vi "App_ShowAppInfo_SplashScreen.vi"() -> ()   [LabVIEW 2014]
panel:
  out "FileDescription":string
  out "LegalCopyright":string
  out "CompanyName":string
  out "InternalName":string
  out "ProductName":string
  out "FileVersion":string
  in  "Close":bool
  # "Application Info"
  # "Version:"
  # "Productname:"
  # "Copyright:"
  # "Company:"
  # "Internal Info:"
  # "FileVersion:"
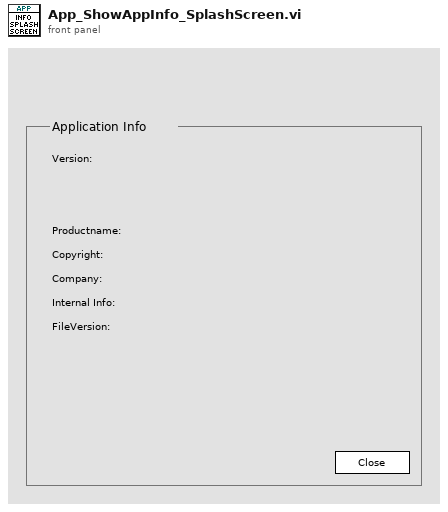
[diagram p1: front panel]
types:
  T1 = enum32{"invalid app kind", "Development System", "Run Time System", "Student Edition", "Embedded LabVIEW", "Evaluation", "Custom"}
  T2 = enum32{"Invalid", "Standard", "Closed", "Hidden", "Minimized", "Maximized"}
  T3 = cluster{"Core":cluster{"Current VI Reference":refnum<vi>, "Close Panel on Exit?":bool}, "Your Boolean data":bool, "Your string data":string}
  T4 = cluster{"Current VI Reference":refnum<vi>, "Close Panel on Exit?":bool}
  T5 = typedef "FileVersionInformation.ctl" = cluster{"FileVersion":string, "ProductName":string, "InternalName":string, "CompanyName":string, "LegalCopyright":string, "FileDescription":string}
  T6 = typedef "SVN_Info_Cluster.ctl" = cluster{"entry.path":string, "entry.revision (HEAD)":i32, "entry.kind":string, "SVN_Log_Cluster":T7}
  T7 = typedef "SVN_LogEntry_Cluster.ctl" = cluster{"revision":i32, "Author":string, "Datetime":timestamp, "Message":string}
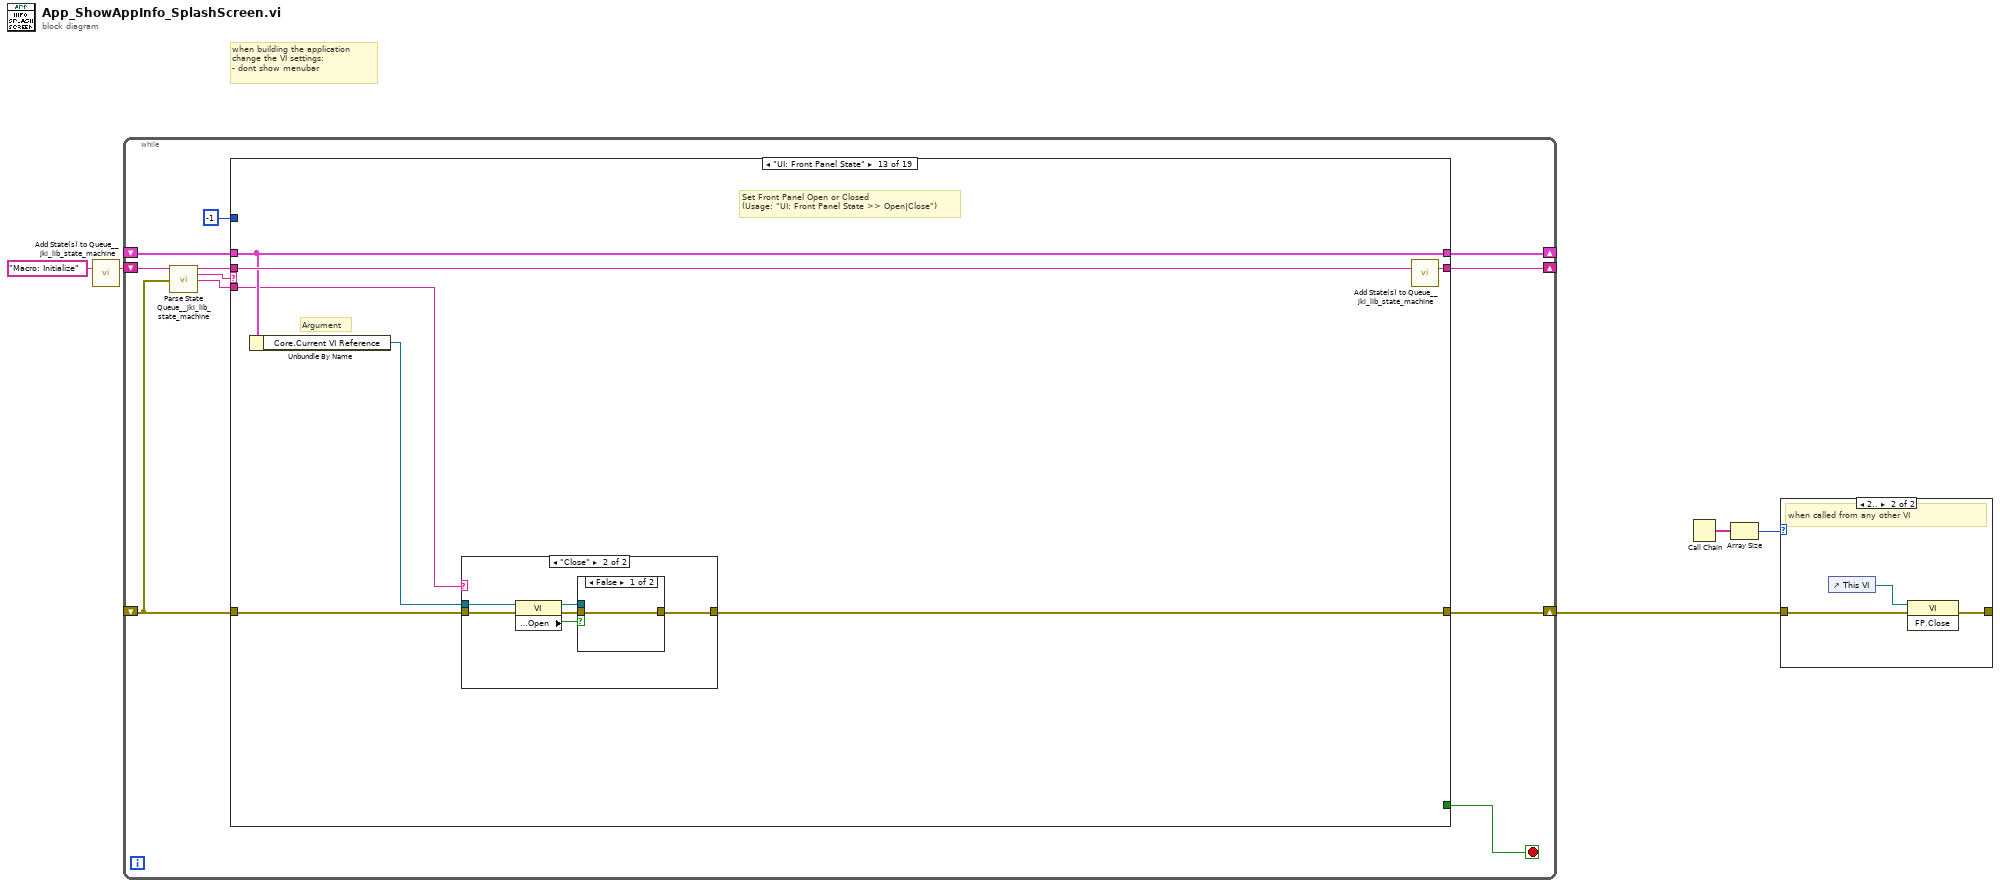
[diagram p0: block diagram]
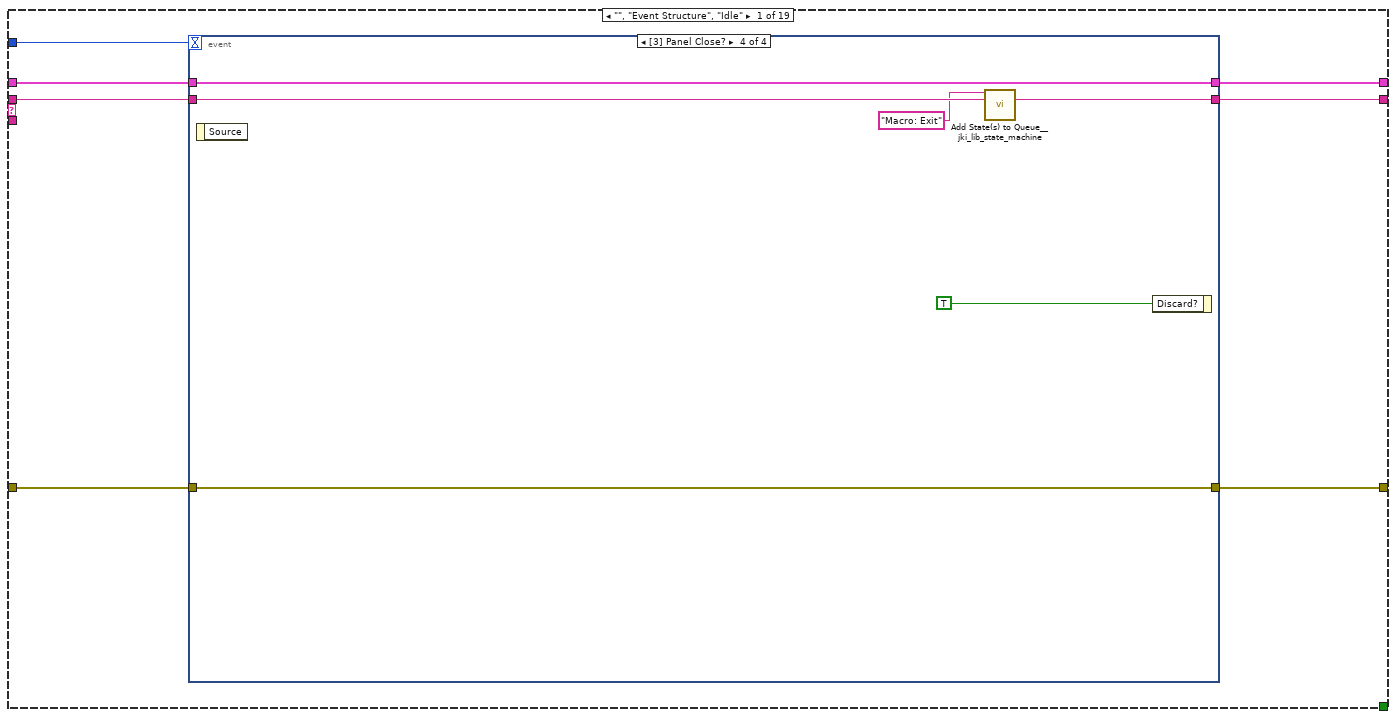
[diagram p3: hidden frame]
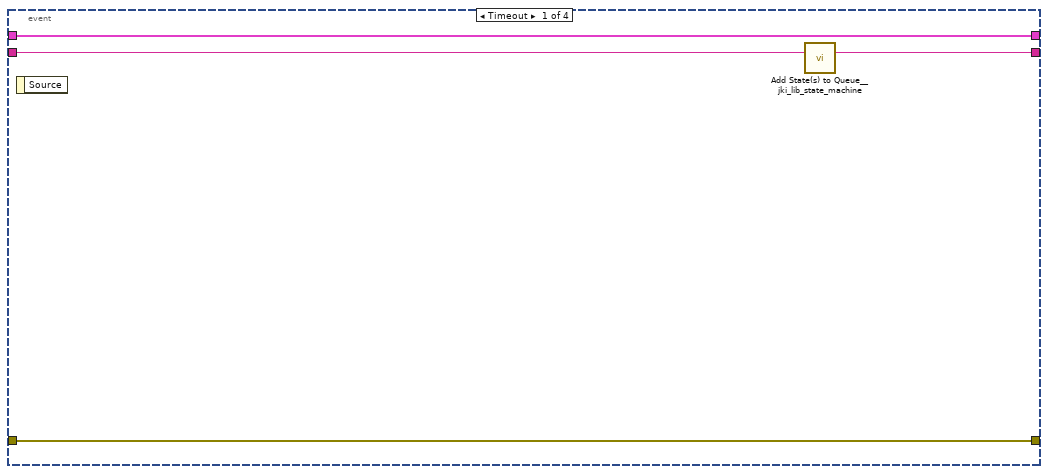
[diagram p4: hidden frame]
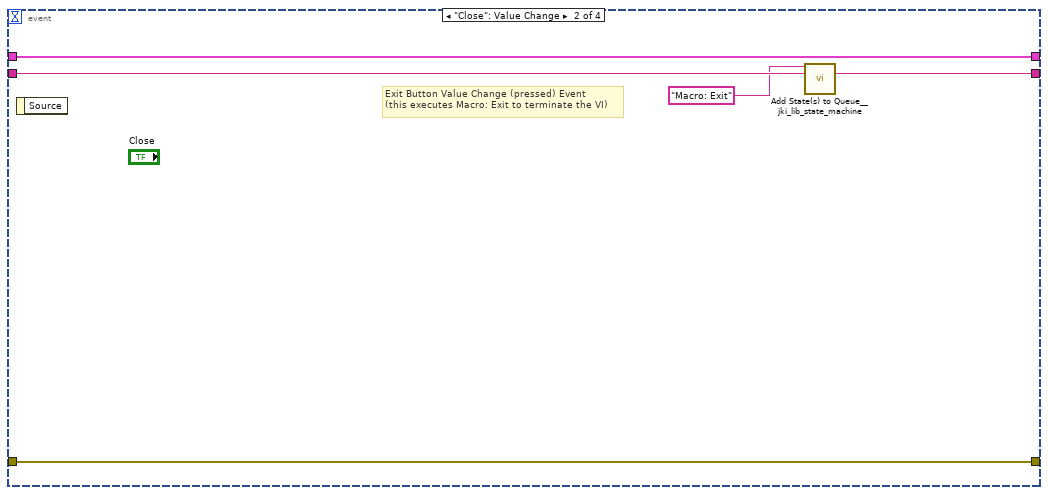
[diagram p5: hidden frame]
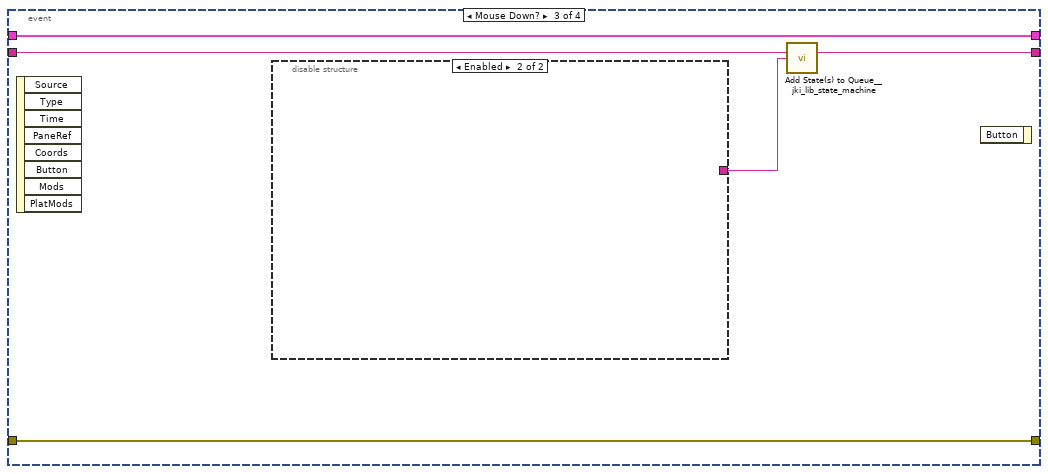
[diagram p6: hidden frame]
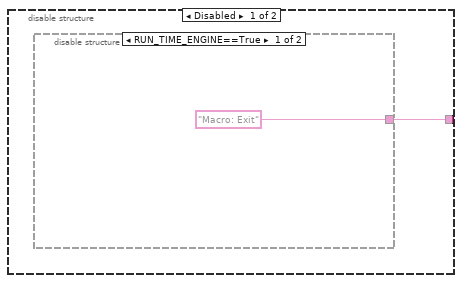
[diagram p7: hidden frame]
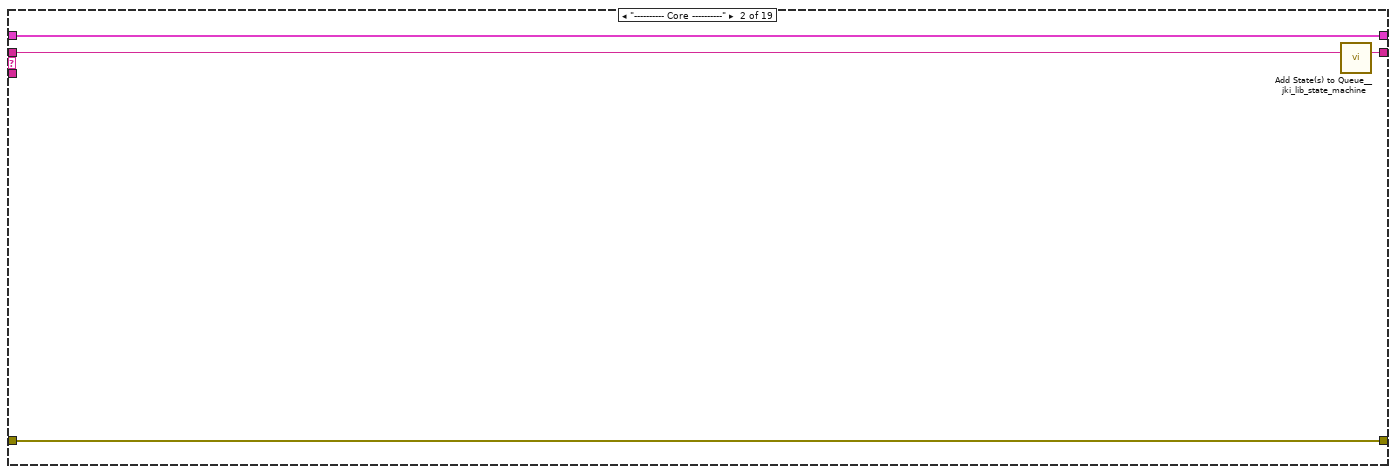
[diagram p9: hidden frame]
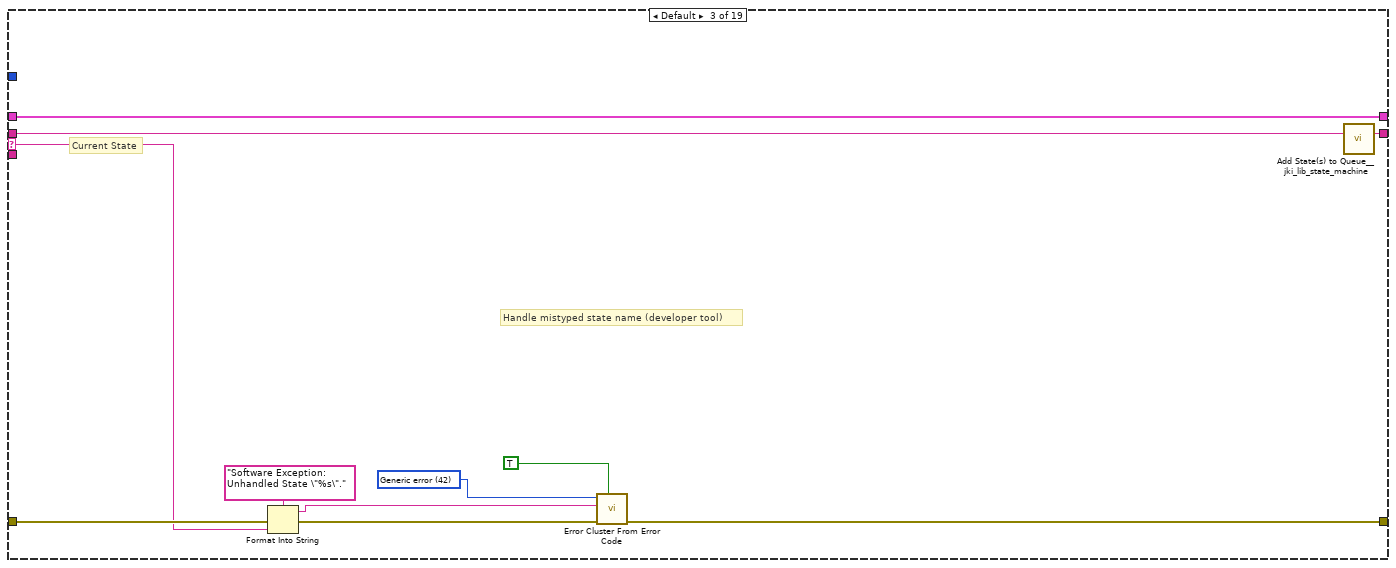
[diagram p10: hidden frame]
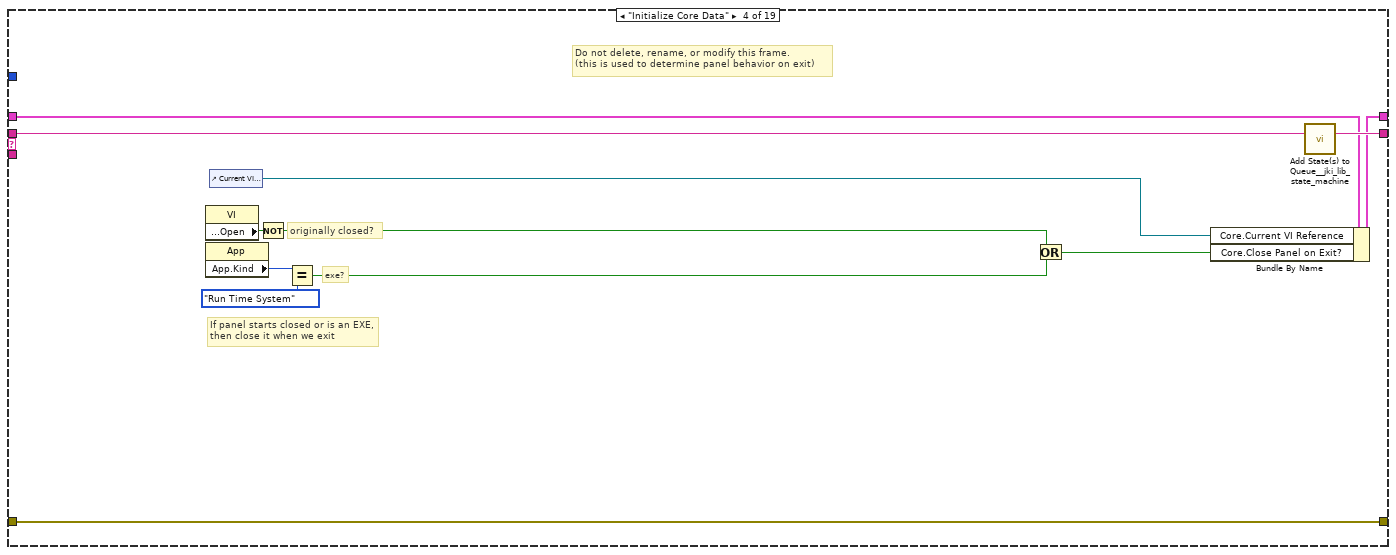
[diagram p11: hidden frame]
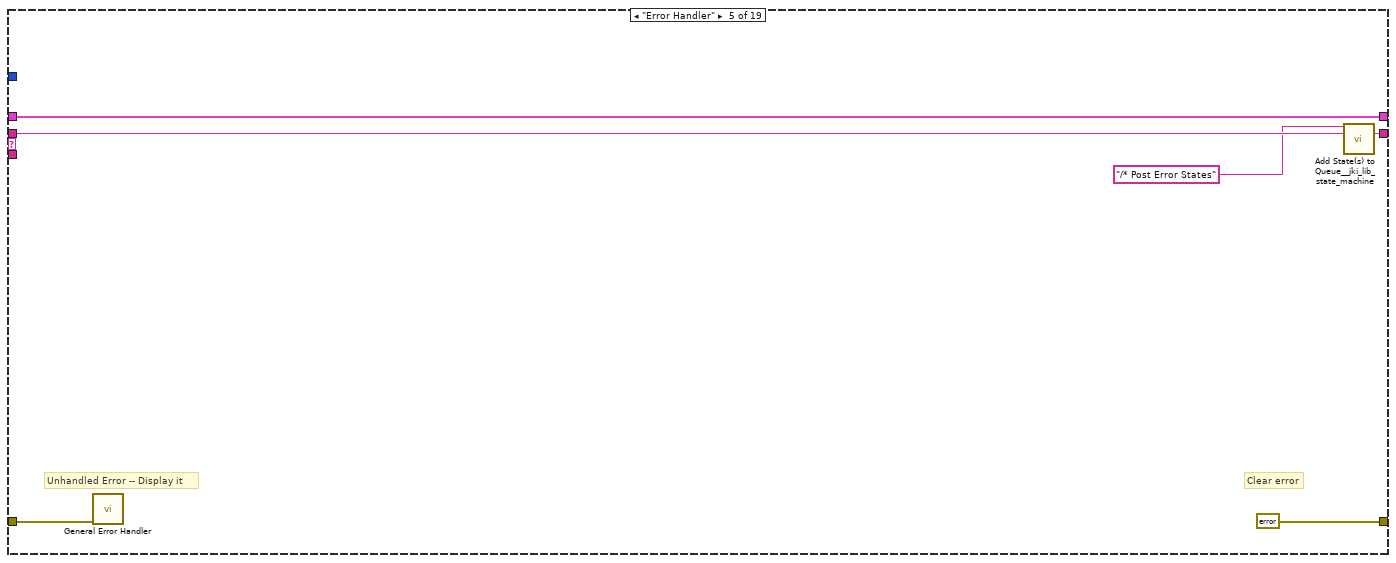
[diagram p12: hidden frame]
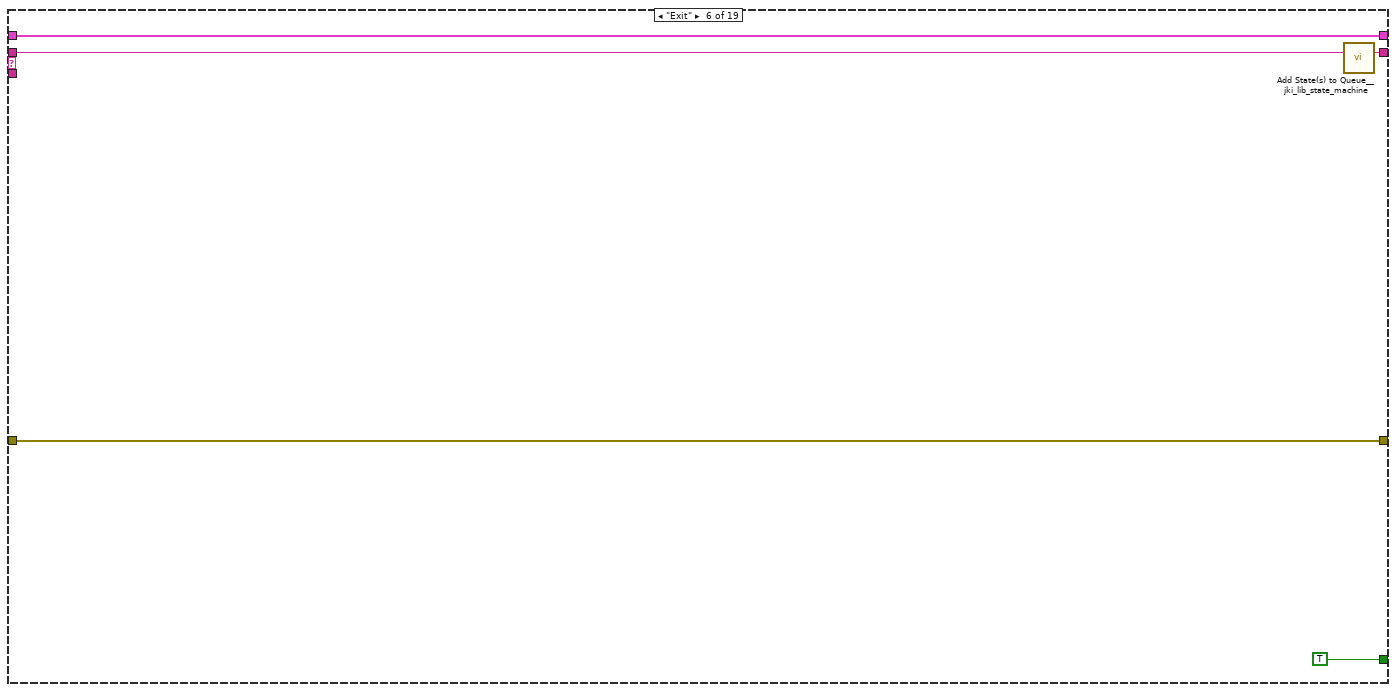
[diagram p13: hidden frame]
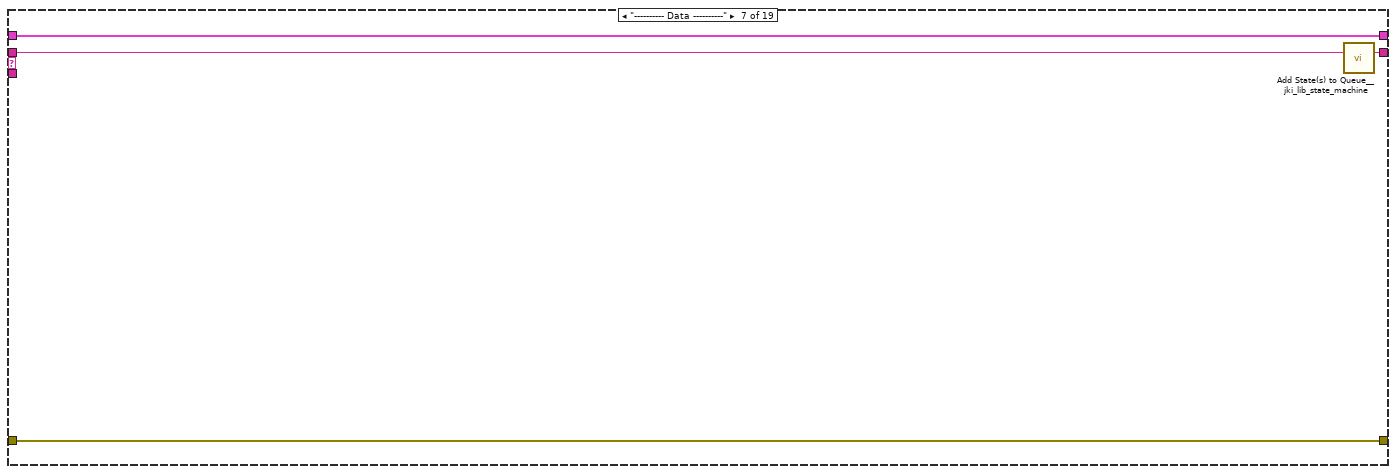
[diagram p14: hidden frame]
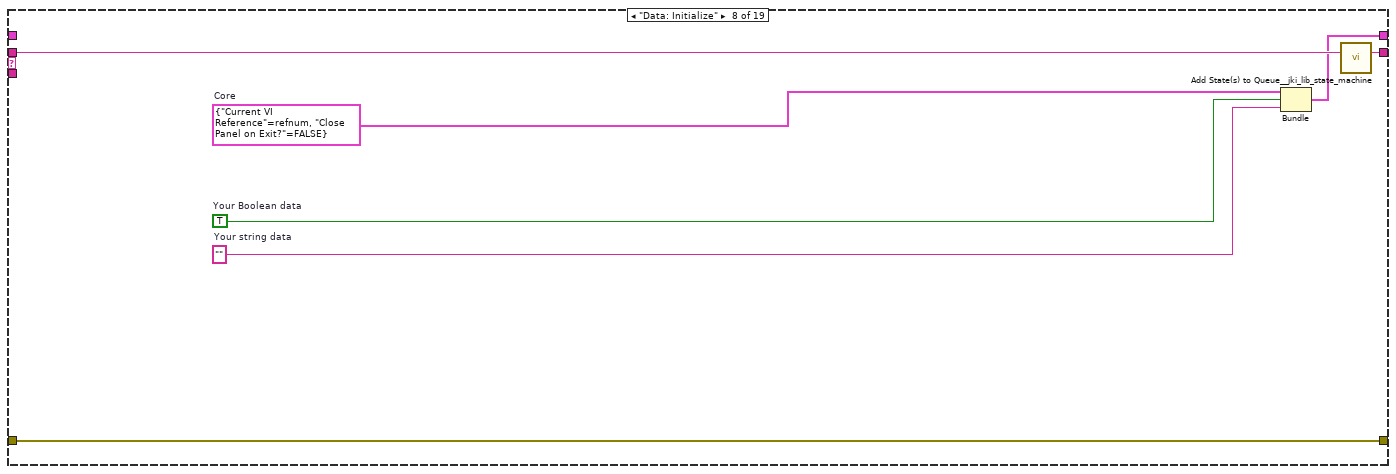
[diagram p15: hidden frame]
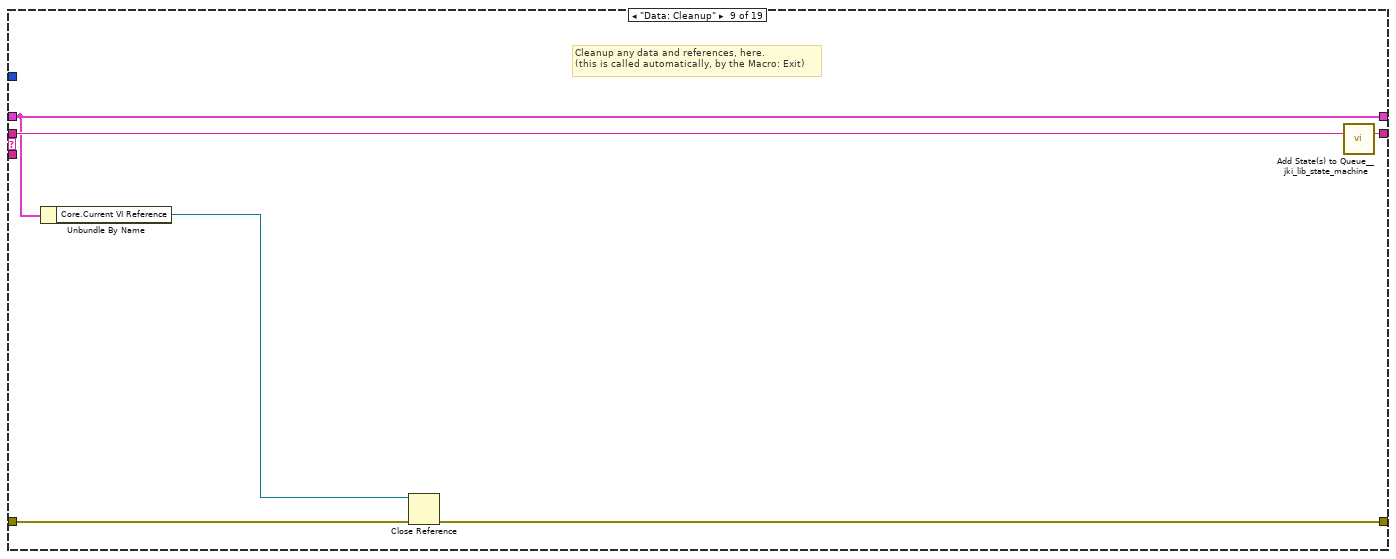
[diagram p16: hidden frame]
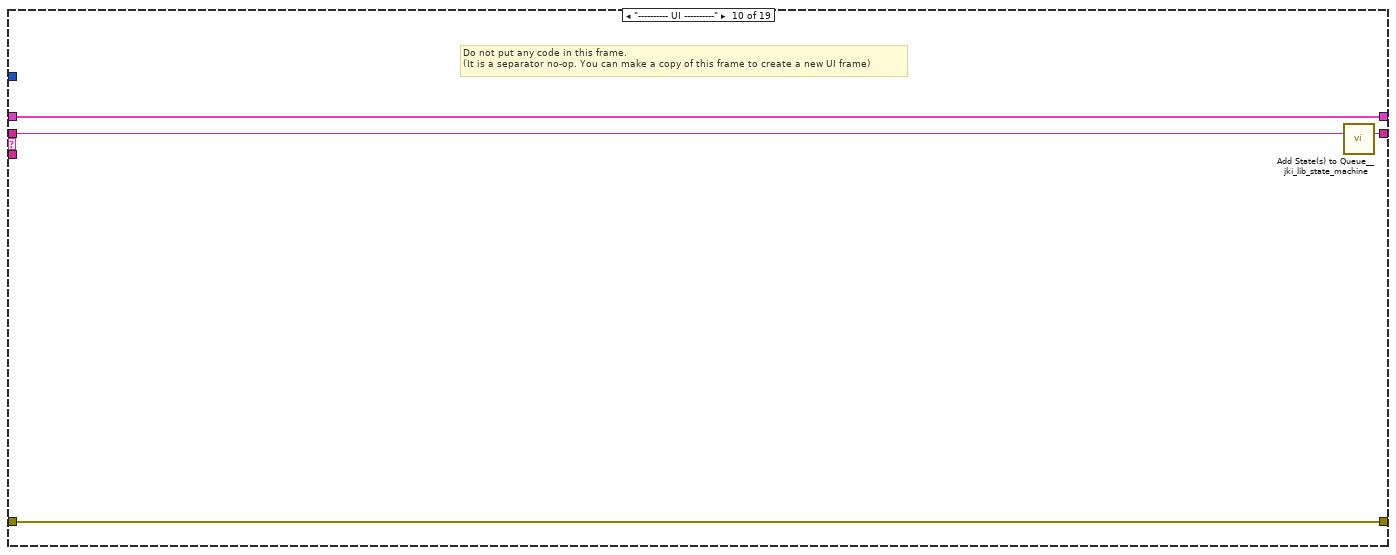
[diagram p17: hidden frame]
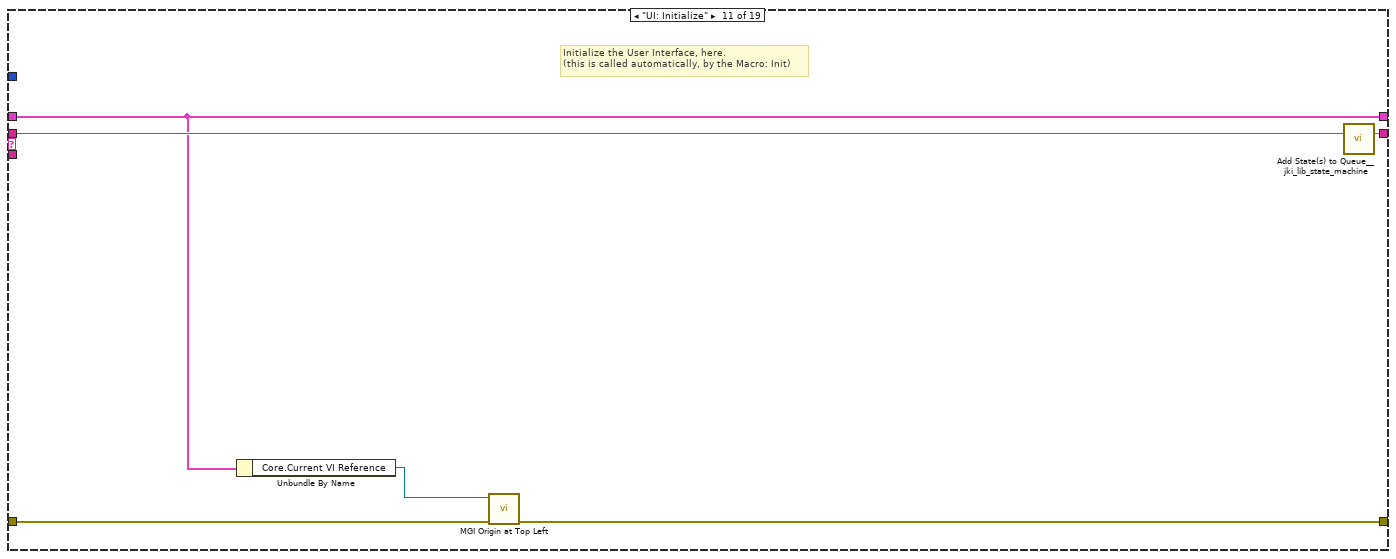
[diagram p18: hidden frame]
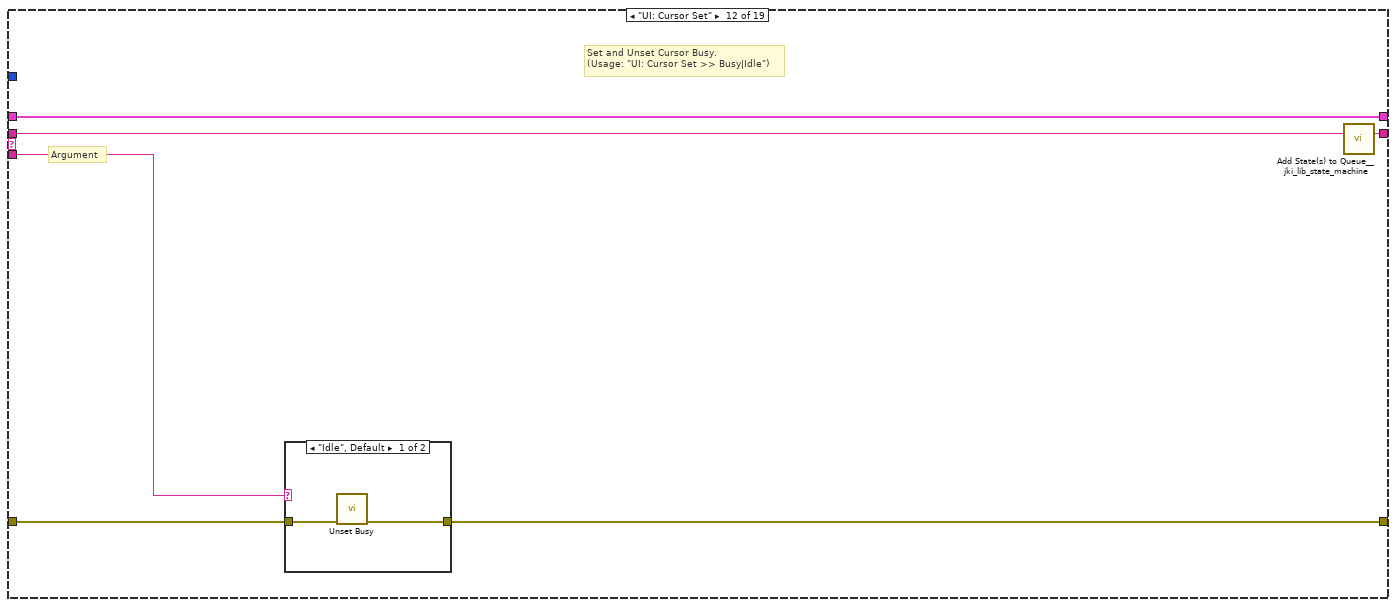
[diagram p19: hidden frame]
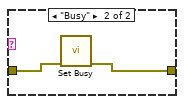
[diagram p20: hidden frame]
diagram:
  # "when building the application\nchange the VI settings:\n- dont show menubar"
  n1 = call <vilib>:"Add State(s) to Queue__jki_lib_state_machine.vi"("State(s) in (\"\")"="Macro: Initialize") -> ("States Out"=w5:string)  [unwired: 14 in]
  n2 = while {
    shift-right: [w9] -> _
    shift-left: _ -> [w8]
    shift-right: [w12] -> w3
    shift-left: _ -> [w6]
    shift-right: [w11] -> _
    shift-left: w5 -> [w13]
    stop <- w10 stop-if-true
    n3 = call <vilib>:"Parse State Queue__jki_lib_state_machine.vi"("State Queue"=w13, "Error In (no error)"=w6) -> ("Remaining States"=w15:string, "Current State"=w16:string, "Arguments"=w14:string)  [unwired: 11 in]
    n4 = case shown="\"UI: Front Panel State\"" w16 {
      selector: w16 -> [_ _ w50 _ _ _ _ _ _ _ _ _ _ _ _ _ _ _ _]
      tunnel: w15 -> [w23 w49 w54 w72 w78 w83 w87 w94 w100 w104 w110 w116 w127 w153 w158 w168 w172 w202 w206]
      tunnel: w14 -> [_ _ _ _ _ _ _ _ _ _ _ w111 w121 _ _ _ _ _ _]
      tunnel: w8 -> [w21 w46 w52 w63 w75 w81 w84 _ w95 w101 w106 w114 w123 w150 w155 w165 w169 w197 w203]
      tunnel: [w20 w47 w56 w69 errorcluster {"status"=FALSE, "code"=0, "source"=""} ("error out") w80 w85 w91 w96 w102 w108 w112 w124 w151 w156 w166 w170 w180 w204] -> w12
      tunnel: w6 -> [w19 w47 w55 w69 w74 w80 w85 w91 w97 w102 w107 w113 w125 w151 w156 w166 w170 w188 w204]
      tunnel: [w22 w48 w53 w71 w77 w82 w86 w93 w99 w103 w109 w115 w126 w152 w157 w167 w171 w201 w205] -> w11
      tunnel: [_ _ _ _ _ TRUE _ _ _ _ _ _ _ _ _ _ _ _ _] -> w10
      tunnel: [w18 w46 w52 w70 w75 w81 w84 w92 w95 w101 w106 w114 w123 w150 w155 w165 w169 w197 w203] -> w9
      tunnel: -1 ("Timeout") -> [w17 _ _ _ _ _ _ _ _ _ _ _ _ _ _ _ _ _ _]
      frame "", "Event Structure", "Idle" {
        n5 = event shown="[3] Panel Close?" {
          selector: _ -> [_ _ _ _]
          dyn-events: _ -> [_ _ _ _]
          timeout: w17 -> [_ _ _ _]
          tunnel: w23 -> [w27 w32 w34 w45]
          tunnel: [w26 w31 w35 w44] -> w22
          tunnel: w21 -> [w24 w29 w36 w42]
          tunnel: [w25 w30 w37 w43] -> w20
          tunnel: w19 -> [w25 w30 w37 w43]
          tunnel: [w24 w29 w36 w42] -> w18
          event Timeout {
            n6 = event-data() -> ()  [unwired: 1 in, 1 out]
            n7 = call <vilib>:"Add State(s) to Queue__jki_lib_state_machine.vi"("State(s) in (\"\")"=w27) -> ("States Out"=w26:string)  [unwired: 14 in]
          }
          event "Close": Value Change {
            # "Exit Button Value Change (pressed) Event\n(this executes Macro: Exit to terminate the VI)"
            n8 = event-data() -> ()  [unwired: 1 in, 1 out]
            n9 = call <vilib>:"Add State(s) to Queue__jki_lib_state_machine.vi"("State(s) in Front (\"\")"="Macro: Exit", "State(s) in (\"\")"=w32) -> ("States Out"=w31:string)  [unwired: 13 in]
          }
          event Mouse Down? {
            n10 = event-data() -> ()  [unwired: 1 in, 8 out]
            n11 = disable-structure shown="Enabled" {
              disable-tunnel: [w38 _] -> w33
              frame Disabled {
                n12 = disable-structure shown="RUN_TIME_ENGINE==True" {
                  disable-tunnel: ["Macro: Exit" _] -> w38
                  frame condition #0 {
                  }
                  frame condition #1 (active) {
                  }
                }
              }
              frame Enabled {
              }
            }
            n13 = call <vilib>:"Add State(s) to Queue__jki_lib_state_machine.vi"("State(s) in (\"\")"=w34, "State(s) at Back (\"\")"=w33) -> ("States Out"=w35:string)  [unwired: 13 in]
            n14 = event-data() -> ()  [unwired: 2 in, 1 out]
          }
          event Panel Close? {
            n15 = event-data() -> ()  [unwired: 1 in, 1 out]
            n16 = call <vilib>:"Add State(s) to Queue__jki_lib_state_machine.vi"("State(s) in Front (\"\")"="Macro: Exit", "State(s) in (\"\")"=w45) -> ("States Out"=w44:string)  [unwired: 13 in]
            n17 = event-data("Discard?"=TRUE) -> ()  [unwired: 1 in, 1 out]
          }
        }
      }
      frame "---------- Core ----------" {
        n18 = call <vilib>:"Add State(s) to Queue__jki_lib_state_machine.vi"("State(s) in (\"\")"=w49) -> ("States Out"=w48:string)  [unwired: 14 in]
      }
      frame Default {
        w59 = 42 items=["No error", "Argument error", "Memory is full", "Out of zone", "End of file", "File already open", "Generic file I/O error", "File not found", "File permission error", "Disk is full", "Duplicate path", "Too many files open", "System feature not enabled", "Resource file not found", "Cannot add resource", "Resource not found", "Image not found", "Image memory error", "Pen does not exist", "Config type invalid", "Config token not found", "Config parse error", "Config memory error", "Bad external code format", "Bad external code offset", "External code not present", "Null window", "Destroy window error", "Null menu", "Print aborted", "Bad print record", "Print driver error", "Windows error during printing", "Memory error during printing", "Print dialog error", "Generic print error", "Invalid device refnum", "Device not found", "Device parameter error", "Device unit error", "Cannot open device", "Device call aborted", "Generic error", "Cancelled by user", "Object ID too low", "Object ID too high", "Object not in heap", "Unknown heap", "Unknown object (invalid DefProc)", "Unknown object (DefProc not in table)", "Message out of range", "Invalid (null) method", "Unknown message", "Manager call not supported", "Bad address", "Network operation in progress", "Network operation timed out", "Connection is busy", "Network attribute not supported", "Network error", "Address in use", "System out of memory", "Connection aborted", "Connection refused", "Not connected", "Already connected", "Connection closed", "Initialization error (interapplication manager)", "Bad occurrence", "Wait on unbound occurrence handler", "Occurrence queue overflow", "Datalog type conflict", "Unused", "Unrecognized type (interapplication manager)", "Memory corrupt", "Failed to make temporary DLL", "Old CIN version", "Drag socket not found", "Failed to load drop-object", "Failed to register OLE object", "Failed to release OLE object", "Format specifier type mismatch", "Unknown format specifier", "Too few format specifiers", "Too many format specifiers", "Scan failed", "Newer CIN version", "Error converting to variant", "Runtime menu error", "Password tampered", "Variant attribute not found", "Incompatible variant data type", "Event data is not available", "Event Store is not present", "Occurrence is not found", "Event Queue is not created", "Event info is not available", "Refnum passed is NULL", "Error retrieving Class GUID", "Error retrieving CoClass GUID", "Error retrieving TypeLib GUID.", "Bad built application magic bytes.", "Specific driver is different from the specific driver associated with the Logical Name.", "There is no session opened to the class driver.", "Max Error", "MAX - Error with config objects", "MAX - Error loading configuration", "MAX - Group not supported"]
        # "Current State"
        # "Handle mistyped state name (developer tool)"
        n19 = Format Into String(format string="Software Exception: Unhandled State \"%s\"." ("message"), error in=w55, w50) -> (resulting string=w58:string, error out=w57:errorcluster)  [unwired: 1 in]
        n20 = call <vilib>:"Error Cluster From Error Code.vi"("show call chain? (False)"=TRUE, "error in (no error)"=w57, "error message (\"\")"=w58, "error code (0)"=w59) -> ("error out"=w56:errorcluster)  [unwired: 5 in]
        n21 = call <vilib>:"Add State(s) to Queue__jki_lib_state_machine.vi"("State(s) in (\"\")"=w54) -> ("States Out"=w53:string)  [unwired: 14 in]
      }
      frame "Initialize Core Data" {
        # "Do not delete, rename, or modify this frame.\n(this is used to determine panel behavior on exit)"
        # "originally closed?"
        # "exe?"
        # "If panel starts closed or is an EXE, then close it when we exit"
        n22 = property class="VI"() -> ("Front Panel.Open"=w68:bool)  [unwired: 2 in, 2 out]
        n23 = property class="App"() -> ("App.Kind"=w67:T1)  [unwired: 2 in, 2 out]
        n24 = control-ref of="Current VI Reference"() -> (w61:refnum<vi>)
        n25 = Not(x=w68) -> (.not. x?=w65:bool)
        n26 = Equal?(x=w67, y=T1."Run Time System" ("Application:Kind")) -> (x = y?=w64:bool)
        n27 = Or(x=w65, y=w64) -> (x .or. y?=w62:bool)
        n28 = Bundle By Name(cluster=w63, "Core.Current VI Reference"=w61, "Core.Close Panel on Exit?"=w62) -> (w70:T3)
        n29 = call <vilib>:"Add State(s) to Queue__jki_lib_state_machine.vi"("State(s) in (\"\")"=w72) -> ("States Out"=w71:string)  [unwired: 14 in]
      }
      frame "Error Handler" {
        # "Unhandled Error -- Display it"
        # "Clear error"
        n30 = call <vilib>:"General Error Handler.vi"("error in (no error)"=w74) -> ()  [unwired: 10 in, 5 out]
        n31 = call <vilib>:"Add State(s) to Queue__jki_lib_state_machine.vi"("State(s) in Front (\"\")"="/* Post Error States", "State(s) in (\"\")"=w78) -> ("States Out"=w77:string)  [unwired: 13 in]
      }
      frame "Exit" {
        n32 = call <vilib>:"Add State(s) to Queue__jki_lib_state_machine.vi"("State(s) in (\"\")"=w83) -> ("States Out"=w82:string)  [unwired: 14 in]
      }
      frame "---------- Data ----------" {
        n33 = call <vilib>:"Add State(s) to Queue__jki_lib_state_machine.vi"("State(s) in (\"\")"=w87) -> ("States Out"=w86:string)  [unwired: 14 in]
      }
      frame "Data: Initialize" {
        w88 = T4 {"Current VI Reference"=refnum, "Close Panel on Exit?"=FALSE}  # Core
        w90 = TRUE  # Your Boolean data
        w89 = ""  # Your string data
        n34 = Bundle("Core"=w88, "Your Boolean data"=w90, "Your string data"=w89) -> (w92:T3)  [unwired: 1 in]
        n35 = call <vilib>:"Add State(s) to Queue__jki_lib_state_machine.vi"("State(s) in (\"\")"=w94) -> ("States Out"=w93:string)  [unwired: 14 in]
      }
      frame "Data: Cleanup" {
        # "Cleanup any data and references, here.\n(this is called automatically, by the Macro: Exit)"
        n36 = Unbundle By Name(w95) -> ("Core.Current VI Reference"=w98:refnum<vi>)
        n37 = Close Reference(reference=w98, error in (no error)=w97) -> (error out=w96:errorcluster)
        n38 = call <vilib>:"Add State(s) to Queue__jki_lib_state_machine.vi"("State(s) in (\"\")"=w100) -> ("States Out"=w99:string)  [unwired: 14 in]
      }
      frame "---------- UI ----------" {
        # "Do not put any code in this frame.\n(It is a separator no-op. You can make a copy of this frame to create a new UI frame)"
        n39 = call <vilib>:"Add State(s) to Queue__jki_lib_state_machine.vi"("State(s) in (\"\")"=w104) -> ("States Out"=w103:string)  [unwired: 14 in]
      }
      frame "UI: Initialize" {
        # "Initialize the User Interface, here.\n(this is called automatically, by the Macro: Init)"
        n40 = Unbundle By Name(w106) -> ("Core.Current VI Reference"=w105:refnum<vi>)
        n41 = call <userlib>:"MGI Origin at Top Left.vi"("Error In"=w107, "VI Reference In (Caller)"=w105) -> ("Error Out"=w108:errorcluster)  [unwired: 7 in, 1 out]
        n42 = call <vilib>:"Add State(s) to Queue__jki_lib_state_machine.vi"("State(s) in (\"\")"=w110) -> ("States Out"=w109:string)  [unwired: 14 in]
      }
      frame "UI: Cursor Set" {
        # "Argument"
        # "Set and Unset Cursor Busy.\n(Usage: \"UI: Cursor Set >> Busy|Idle\")"
        n43 = case shown="\"Idle\", Default" w111 {
          tunnel: w113 -> [w118 w120]
          tunnel: [w117 w119] -> w112
          frame "Idle", Default {
            n44 = call <vilib>:"Unset Busy.vi"("error in (no error)"=w118) -> ("error out"=w117:errorcluster)  [unwired: 10 in]
          }
          frame "Busy" {
            n45 = call <vilib>:"Set Busy.vi"("error in (no error)"=w120) -> ("error out"=w119:errorcluster)  [unwired: 9 in, 1 out]
          }
        }
        n46 = call <vilib>:"Add State(s) to Queue__jki_lib_state_machine.vi"("State(s) in (\"\")"=w116) -> ("States Out"=w115:string)  [unwired: 14 in]
      }
      frame "UI: Front Panel State" {
        # "Argument"
        # "Set Front Panel Open or Closed\n(Usage: \"UI: Front Panel State >> Open|Close\")"
        n47 = Unbundle By Name(w123) -> ("Core.Current VI Reference"=w122:refnum<vi>)
        n48 = case shown="\"Close\"" w121 {
          tunnel: w125 -> [w131 w144]
          tunnel: [w133 w145] -> w124
          tunnel: w122 -> [w132 w142]
          frame "Open", Default {
            n49 = property class="VI"(reference=w132, error in=w131) -> (reference out=w129:refnum<vi>, error out=w130:errorcluster, "Front Panel.Open"=w128:bool)
            n50 = case shown="False" w128 {
              tunnel: [w136 w139] -> w133
              tunnel: w130 -> [w135 w139]
              tunnel: w129 -> [w134 _]
              frame False {
                n51 = invoke class="VI" method="FP.Open"(reference=w134, error in=w135, "Activate"=TRUE, "State"=T2."Standard") -> (error out=w136:errorcluster)  [unwired: 1 in, 4 out]
              }
              frame True {
              }
            }
          }
          frame "Close" {
            n52 = property class="VI"(reference=w142, error in=w144) -> (reference out=w141:refnum<vi>, error out=w143:errorcluster, "Front Panel.Open"=w140:bool)
            n53 = case shown="False" w140 {
              tunnel: [w146 w149] -> w145
              tunnel: w143 -> [w146 w148]
              tunnel: w141 -> [_ w147]
              frame False {
              }
              frame True {
                n54 = invoke class="VI" method="FP.Close"(reference=w147, error in=w148) -> (error out=w149:errorcluster)  [unwired: 1 in, 2 out]
              }
            }
          }
        }
        n55 = call <vilib>:"Add State(s) to Queue__jki_lib_state_machine.vi"("State(s) in (\"\")"=w127) -> ("States Out"=w126:string)  [unwired: 14 in]
      }
      frame "---------- Macro ----------" {
        n56 = call <vilib>:"Add State(s) to Queue__jki_lib_state_machine.vi"("State(s) in (\"\")"=w153) -> ("States Out"=w152:string)  [unwired: 14 in]
      }
      frame "Macro: Initialize" {
        w154 = "Data: Initialize\nInitialize Core Data\nUI: Front Panel State >> Close\nUI: Initialize\nAppISS: ShowStats\nUI: Front Panel State >> Open\n"  # Data: Initialize Initialize Core Data UI: Front Panel State >> Close UI: Initialize AppISS: ShowStats UI: Front Panel State >> Open
        n57 = call <vilib>:"Add State(s) to Queue__jki_lib_state_machine.vi"("State(s) in Front (\"\")"=w154, "State(s) in (\"\")"=w158) -> ("States Out"=w157:string)  [unwired: 13 in]
      }
      frame "Macro: Exit" {
        # "Exit Macro\n(This is called once, when the VI exits)"
        n58 = Unbundle By Name(w165) -> ("Core.Close Panel on Exit?"=w164:bool)
        n59 = Select(t="UI: Front Panel State >> Close", s=w164, f="") -> (s? t:f=w161:string)
        n60 = call <vilib>:"Add State(s) to Queue__jki_lib_state_machine.vi"("State(s) in (\"\")"=w161, "State(s) at Back (\"\")"="Data: Cleanup\nExit") -> ("States Out"=w159:string)  [unwired: 13 in]
        n61 = call <vilib>:"Add State(s) to Queue__jki_lib_state_machine.vi"("State(s) in Front (\"\")"=w159, "State(s) in (\"\")"=w168) -> ("States Out"=w167:string)  [unwired: 13 in]
      }
      frame "---------- New Category ----------" {
        # "Template Separator\n(You can make a copy of, or modify, this frame)"
        n62 = call <vilib>:"Add State(s) to Queue__jki_lib_state_machine.vi"("State(s) in (\"\")"=w172) -> ("States Out"=w171:string)  [unwired: 14 in]
      }
      frame "AppISS: ShowStats" {
        w189 = path "L:/Program Files/National Instruments/MyProj - My" ("repo path")
        # "Base"
        # "Head"
        n63 = Unbundle By Name(w197) -> ()  [unwired: 1 out]
        n64 = call "App_GetBuildInfoDevAndRunTime.vi"("Error In"=w188) -> ("Error Out"=w199:errorcluster, "FileVersionInfo Out"=w200:T5)  [unwired: 7 in, 2 out]
        n65 = call "SVN_Info.vi"("rev End"=-2, "Error In"=w188, "repo path"=w189) -> ("Error Out"=w187:errorcluster, "SVN_Info_Cluster"=w185:T6)  [unwired: 7 in]
        n66 = call "SVN_Info.vi"("rev End"=-3, "Error In"=w188, "repo path"=w189) -> ("Error Out"=w186:errorcluster, "SVN_Info_Cluster"=w179:T6)  [unwired: 7 in]
        n67 = Unbundle By Name(w179) -> ("entry.revision (HEAD)"=w176:i32)
        n68 = Unbundle By Name(w185) -> ("SVN_Log_Cluster.revision"=w184:i32)
        n69 = Unbundle By Name(w179) -> ("SVN_Log_Cluster.revision"=w183:i32)
        n70 = Merge Errors(w187, w186) -> (w181:errorcluster)
        n71 = Unbundle By Name(w200) -> ("FileVersion"=w175:string, "ProductName"=w196:string, "InternalName"=→"InternalName":string, "CompanyName"=→"CompanyName":string, "LegalCopyright"=→"LegalCopyright":string, "FileDescription"=→"FileDescription":string)
        "ProductName" <- w196
        n72 = Subtract(x=w184, y=w183) -> ()  [unwired: 1 out]
        n73 = Format Into String(format string="\\nSVN: current repo-revisionnumber: %d", initial string=w175, w176) -> (resulting string=w174:string)  [unwired: 1 in, 1 out]
        n74 = call <userlib>:"MGI Is Runtime.vi"() -> ("Run Time System?"=w178:bool)  [unwired: 7 in]
        n75 = Select(t=w175, s=w178, f=w174) -> (s? t:f=→"FileVersion":string)
        n76 = Unbundle By Name(w197) -> ("Core.Current VI Reference"=w198:refnum<vi>)
        n77 = call <userlib>:"MGI Set Front Panel Title.vi"("Error In"=w199, "Front Panel Window:Title"=w196, "VI Reference In (Caller)"=w198) -> ("Error Out"=w182:errorcluster)  [unwired: 6 in, 1 out]
        n78 = Merge Errors(w182, w181) -> (w180:errorcluster)
        n79 = call <vilib>:"Add State(s) to Queue__jki_lib_state_machine.vi"("State(s) in (\"\")"=w202) -> ("States Out"=w201:string)  [unwired: 14 in]
      }
      frame "New Category: 2" {
        n80 = call <vilib>:"Add State(s) to Queue__jki_lib_state_machine.vi"("State(s) in (\"\")"=w206) -> ("States Out"=w205:string)  [unwired: 14 in]
      }
    }
  }
  n81 = Call Chain() -> (call chain=w2:string[])
  n82 = Array Size(array=w2) -> (size(s)=w1:i32)
  n83 = case shown="2.." w1 {
    tunnel: w3 -> [w207 w209]
    tunnel: [w207 w208] -> _
    frame ..1, Default {
      # "use for debugging"
    }
    frame 2.. {
      # "when called from any other VI"
      n84 = control-ref of="This VI"() -> (w210:refnum<vi>)
      n85 = invoke class="VI" method="FP.Close"(reference=w210, error in=w209) -> (error out=w208:errorcluster)  [unwired: 1 in, 2 out]
    }
  }
